vi "Test Load GIF (Path).vi"(8 "error in (no error)":errorcluster) -> (0 "error out":errorcluster, 3 "Pass?":bool)   [LabVIEW 2020]
uses:
  G-Image/Image IO/Polymorphic VIs/Load Image (Path).vi
  G-Image/G-Image.lvlib
panel:
  out "Array":cluster{string, "new picture":picture}[](array[cluster])
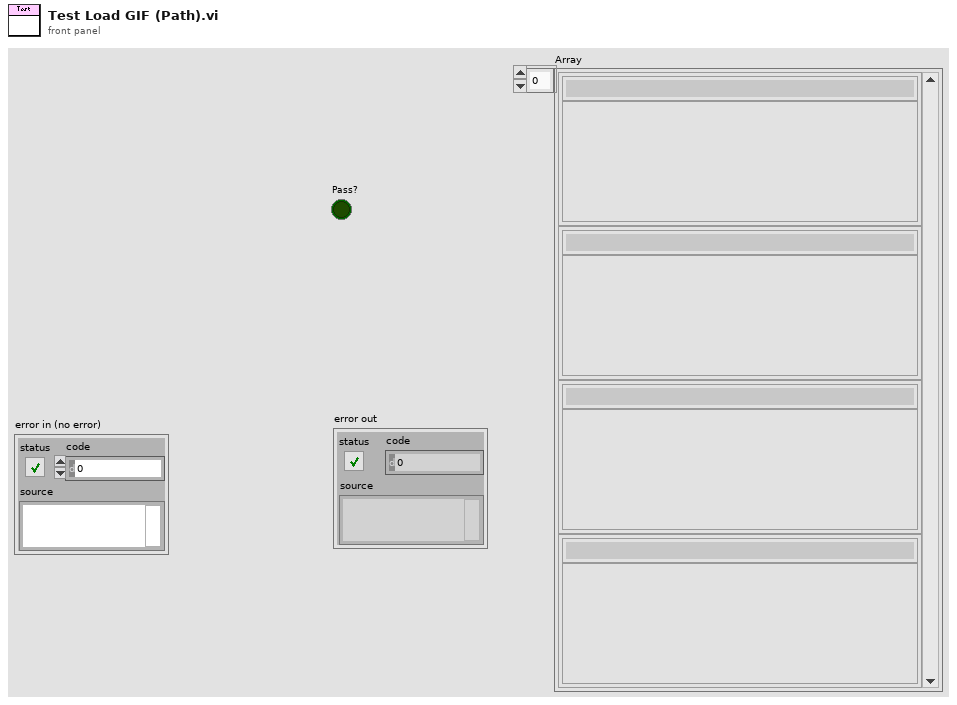
[diagram p1: front panel]
types:
  T1 = typedef "imagedata.ctl" = cluster{"image type":i32, "image depth":i32, "image":u8[], "mask":u8[], "colors":u32[], "Rectangle":cluster{"left":i16, "top":i16, "right":i16, "bottom":i16}}
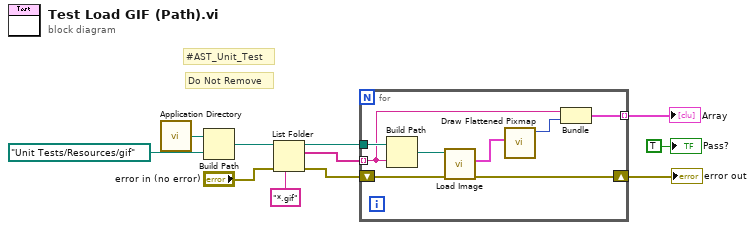
[diagram p0: block diagram]
diagram:
  # "Do Not Remove"
  # "#AST_Unit_Test"
  n1 = call <vilib>:"Application Directory.vi"() -> ("Application Directory"=w11:path)
  n2 = Build Path(base path=w11, name or relative path=path "Unit Tests/Resources/gif" ("Path")) -> (appended path=w9:path)
  n3 = List Folder(path=w9, pattern="*.gif", error in="error in (no error)") -> (path out=w7:path, filenames=w6:string[], error out=w4:errorcluster)  [unwired: 1 in, 1 out]
  n4 = for {
    tunnel: w7 -> [w19]
    tunnel: w6 -> [w13] mode=indexing
    shift-right: [w16] -> w3
    shift-left: w4 -> [w17]
    tunnel: [w12] -> w2 mode=indexing
    n5 = Build Path(base path=w19, name or relative path=w13) -> (appended path=w18:path)
    n6 = call-poly "Load Image.vi"("error in (no error)"=w17, "Path In"=w18) -> ("error out"=w16:errorcluster, "Image"=w15:T1)  [unwired: 7 in, 1 out]
    n7 = call <vilib>:"Draw Flattened Pixmap.vi"("image data"=w15) -> ("new picture"=w14:picture)  [unwired: 8 in]
    n8 = Bundle(w13, "new picture"=w14) -> (w12:cluster{string, "new picture":picture})  [unwired: 1 in]
  }
  "error out" <- w3
  "Array" <- w2
  "Pass?" <- TRUE ("Pass?")
